vi "output.vi"(8 "error in":errorcluster, 10 "data table in":T1, 11 "UI Reference runtime in":refnum<class "io runtime.lvclass">) -> (0 "error out":errorcluster, 2 "data table out":T1, 3 "UI Reference runtime out":refnum<class "io runtime.lvclass">)   [LabVIEW 2015, in "io runtime.lvclass"]
doc: "Provides an interface for writing data to a module at runtime. While this interface performs no operations, a child should provide an override which may write to any open sessions, references, or interfaces."
uses:
  io runtime.lvclass
  <vilib>/NI/Tag Bus/table/data table.ctl
  io runtime.lvclass/io runtime.ctl
  FXP I_20_5.ctl
  FXP I_24_5.ctl
  FXP I_24_10.ctl
  <vilib>/NI/Tag Bus/table/data polymorphs/read many/read Doubles.vi
  <vilib>/NI/Tag Bus/table/data polymorphs/read many/read Singles.vi
  <vilib>/NI/Tag Bus/table/data polymorphs/read many/read I64s.vi
  <vilib>/NI/Tag Bus/table/data polymorphs/read many/read I32s.vi
  <vilib>/NI/Tag Bus/table/data polymorphs/read many/read I16s.vi
  <vilib>/NI/Tag Bus/table/data polymorphs/read many/read I8s.vi
  <vilib>/NI/Tag Bus/table/data polymorphs/read many/read U64s.vi
  <vilib>/NI/Tag Bus/table/data polymorphs/read many/read U32s.vi
  <vilib>/NI/Tag Bus/table/data polymorphs/read many/read U16s.vi
  <vilib>/NI/Tag Bus/table/data polymorphs/read many/read U8s.vi
  <vilib>/NI/Tag Bus/table/data polymorphs/read many/read Booleans.vi
  <vilib>/NI/Tag Bus/table/data polymorphs/read many/read Array of Booleans.vi
  <vilib>/NI/Tag Bus/table/data polymorphs/read one/read Array of Double.vi
  <vilib>/NI/Tag Bus/table/data polymorphs/read one/read Array of Single.vi
  <vilib>/NI/Tag Bus/table/data polymorphs/read one/read Array of I64.vi
  <vilib>/NI/Tag Bus/table/data polymorphs/read one/read Array of I32.vi
  <vilib>/NI/Tag Bus/table/data polymorphs/read one/read Array of I16.vi
  <vilib>/NI/Tag Bus/table/data polymorphs/read one/read Array of I8.vi
  <vilib>/NI/Tag Bus/table/data polymorphs/read one/read Array of U64.vi
  <vilib>/NI/Tag Bus/table/data polymorphs/read one/read Array of U32.vi
  <vilib>/NI/Tag Bus/table/data polymorphs/read one/read Array of U16.vi
  <vilib>/NI/Tag Bus/table/data polymorphs/read one/read Array of U8.vi
  <vilib>/rvi/errors/niLvFpgaAdjustHostInterfaceError.vi
  <vilib>/Utility/error.llb/Error Cluster From Error Code.vi
  <vilib>/rvi/interface/nirviReadWriteControl/nirviReadWriteControl.xnode
  <vilib>/NI/Tag Bus/table/data table.lvlib
  NiFpgaLv.dll
  <vilib>/rvi/interface/Simulation/niFpgaSimulationCallBeginRW.vi
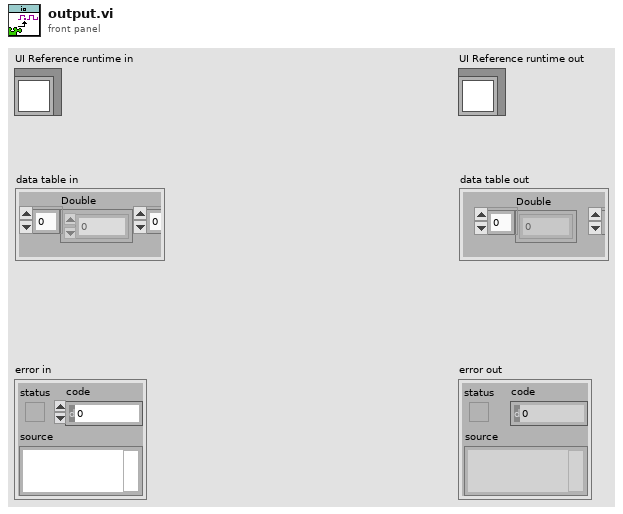
[diagram p1: front panel]
types:
  T1 = typedef "tag bus.lvlib/data table.lvlib/data table.ctl" = cluster{"Double":dbl[], "Single":sgl[], "I64":i64[], "I32":i32[], "I16":i16[], "I8":i8[], "U64":u64[], "U32":u32[], "U16":u16[], "U8":u8[], "Boolean":bool[], "String":string[], "Array of Double":cluster{"DBL Array":dbl[]}[], "Array of Single":cluster{"SGL Array":sgl[]}[], "Array of I64":cluster{"I64 Array":i64[]}[], "Array of I32":cluster{"I32 Array":i32[]}[], "Array of I16":cluster{"I16 Array":i16[]}[], "Array of I8":cluster{"I8 Array":i8[]}[], "Array of U64":cluster{"U64 Array":u64[]}[], "Array of U32":cluster{"U32 Array":u32[]}[], "Array of U16":cluster{"U16 Array":u16[]}[], "Array of U8":cluster{"U8 Array":u8[]}[], "Array of Boolean":cluster{"Boolean Array":bool[]}[], "Array of String":cluster{"String Array":string[]}[]}
  T2 = typedef "io runtime.lvclass/control index set.ctl" = cluster{"data type":T3, "fpga res type":T4[], "fpga resource":refnum<k20>[], "data indexes":i32[], "fifo timeout":refnum<k20>[], "fifo reset":refnum<k20>[], "fifo average":i32[], "fifo samples":u32[], "fifo channels":u32[]}
  T3 = typedef "tag bus.lvlib/tag descriptor.lvclass/Data Type.ctl" = enum16{"Double", "Single", "I64", "I32", "I16", "I8", "U64", "U32", "U16", "U8", "Boolean", "String", "Array of Double", "Array of Single", "Array of I64", "Array of I32", "Array of I16", "Array of I8", "Array of U64", "Array of U32", "Array of U16", "Array of U8", "Array of Boolean", "Array of String"}
  T4 = typedef "io configuration.lvclass/fpga resource supported data types.ctl" = enum16{"Invalid Type", "Single", "I64", "I32", "I16", "I8", "U64", "U32", "U16", "U8", "Boolean", "FXP I,20,5", "FXP I,24,5", "FXP I,24,10", "Fifo 1023,I16"}
  T5 = typedef "io runtime.lvclass/FXP I_20_5.ctl" = refnum<k20>
  T6 = typedef "io runtime.lvclass/FXP I_24_5.ctl" = refnum<k20>
  T7 = typedef "io runtime.lvclass/FXP I_24_10.ctl" = refnum<k20>
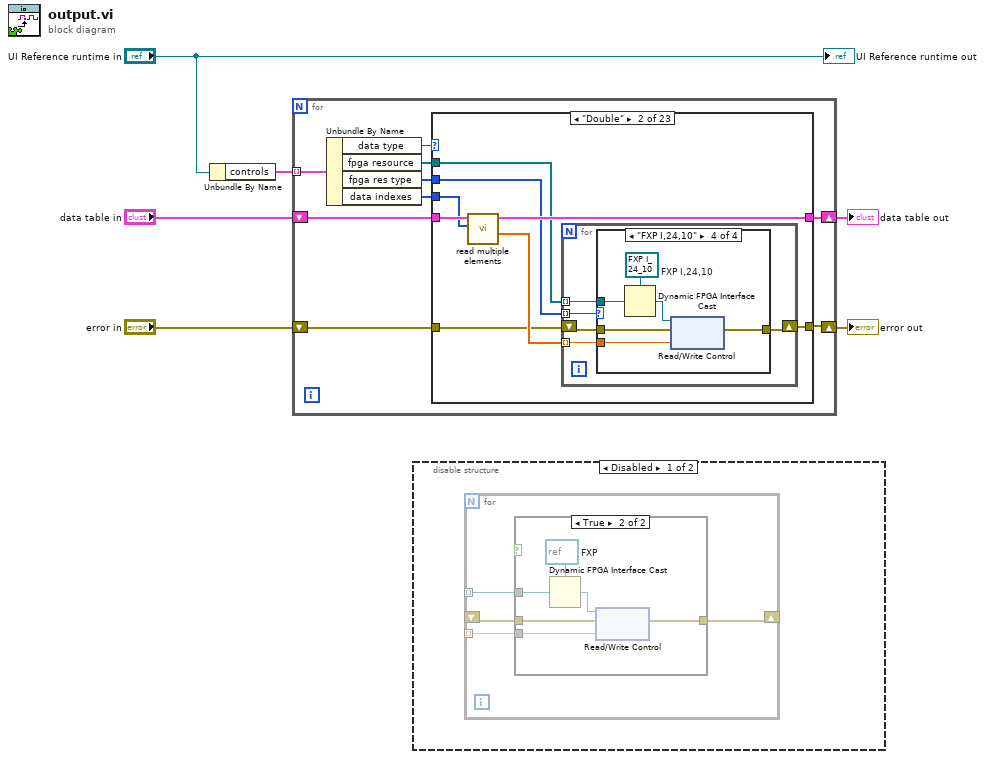
[diagram p0: block diagram]
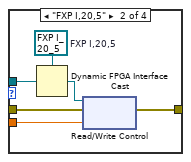
[diagram p6: hidden frame]
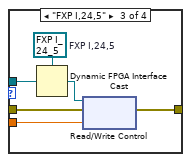
[diagram p7: hidden frame]
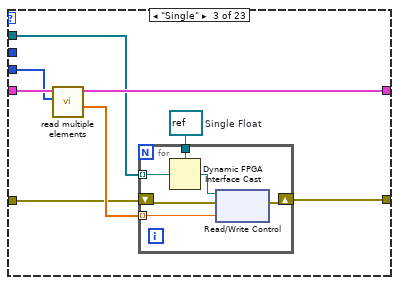
[diagram p8: hidden frame]
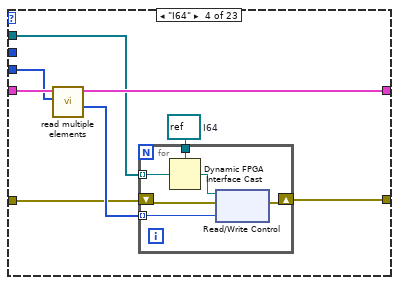
[diagram p9: hidden frame]
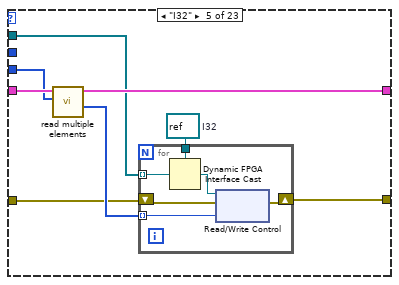
[diagram p10: hidden frame]
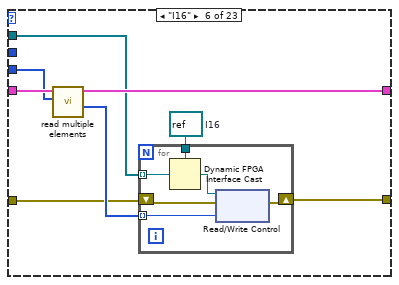
[diagram p11: hidden frame]
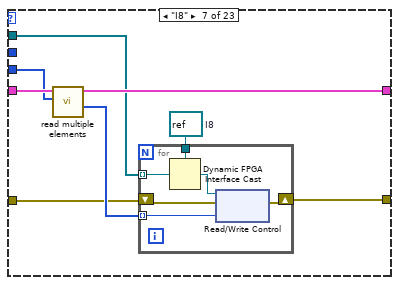
[diagram p12: hidden frame]
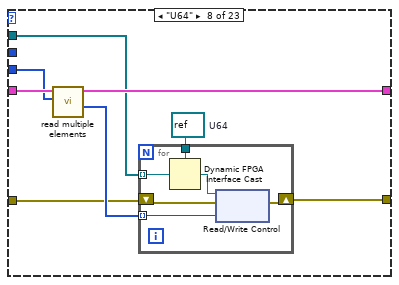
[diagram p13: hidden frame]
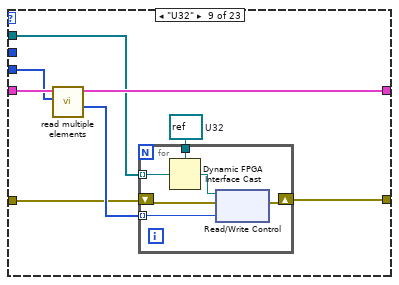
[diagram p14: hidden frame]
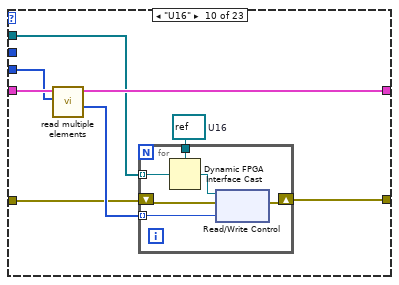
[diagram p15: hidden frame]
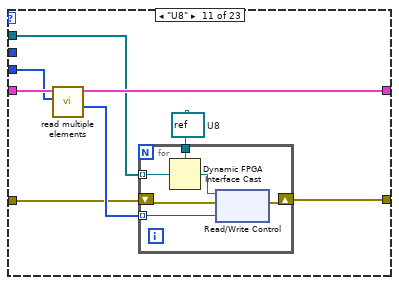
[diagram p16: hidden frame]
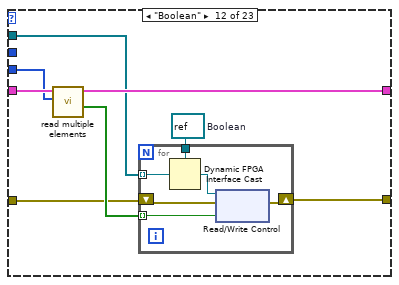
[diagram p17: hidden frame]
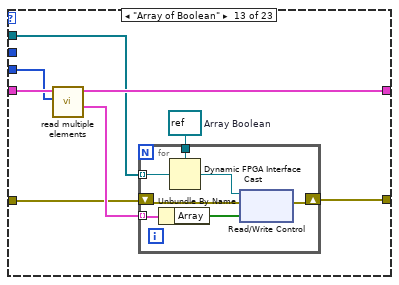
[diagram p18: hidden frame]
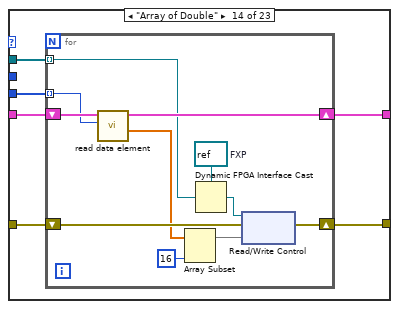
[diagram p19: hidden frame]
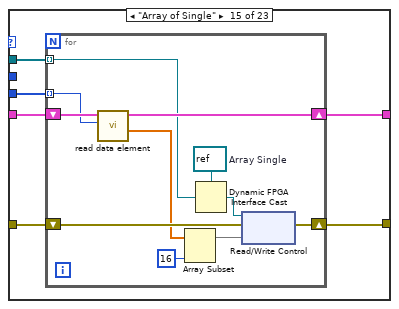
[diagram p20: hidden frame]
diagram:
  n1 = Unbundle By Name("UI Reference runtime in") -> ("controls"=w6:T2[])
  n2 = for {
    shift-right: [w14] -> w2
    shift-left: "data table in" -> [w13]
    shift-right: [w9] -> w4
    shift-left: "error in" -> [w12]
    tunnel: w6 -> [w15] mode=indexing
    n3 = Unbundle By Name(w15) -> ("data type"=w8:T3, "fpga resource"=w10:refnum<k20>[], "fpga res type"=w7:T4[], "data indexes"=w11:i32[])
    n4 = case shown="\"Double\"" w8 {
      tunnel: [w17 w24 w56 w70 w84 w98 w112 w126 w140 w154 w168 w182 w196 w209 w226 w243 w260 w276 w293 w310 w327 w344 w361] -> w14
      tunnel: w13 -> [w17 w25 w57 w71 w85 w99 w113 w127 w141 w155 w169 w183 w197 w210 w227 w244 w261 w277 w294 w311 w328 w345 w362]
      tunnel: w12 -> [w16 w21 w53 w67 w81 w95 w109 w123 w137 w151 w165 w179 w193 w207 w224 w241 w258 w274 w291 w308 w325 w342 w359]
      tunnel: w11 -> [_ w23 w55 w69 w83 w97 w111 w125 w139 w153 w167 w181 w195 w208 w225 w242 w259 w275 w292 w309 w326 w343 w360]
      tunnel: w10 -> [_ w20 w52 w66 w80 w94 w108 w122 w136 w150 w164 w178 w192 w206 w223 w240 w257 w273 w290 w307 w324 w341 w358]
      tunnel: [w16 w19 w50 w64 w78 w92 w106 w120 w134 w148 w162 w176 w191 w205 w222 w239 w256 w272 w289 w306 w323 w340 w357] -> w9
      tunnel: w7 -> [_ w18 _ _ _ _ _ _ _ _ _ _ _ _ _ _ _ _ _ _ _ _ _]
      frame Default {
      }
      frame "Double" {
        n5 = call-poly <vilib>:"read multiple elements.vi"("indices"=w23, "data table in"=w25) -> ("values"=w22:dbl[], "data table out"=w24:T1)  [unwired: 8 in]
        n6 = for {
          tunnel: w20 -> [w30] mode=indexing
          shift-right: [w28] -> w19
          shift-left: w21 -> [w29]
          tunnel: w22 -> [w27] mode=indexing
          tunnel: w18 -> [w26] mode=indexing
          n7 = case shown="\"FXP I,24,10\"" w26 {
            tunnel: w30 -> [_ w37 w43 w49]
            tunnel: w29 -> [w31 w35 w41 w47]
            tunnel: [w31 w34 w40 w46] -> w28
            tunnel: w27 -> [_ w33 w39 w45]
            frame "Invalid Type", Default {
            }
            frame "FXP I,20,5" {
              w32 = T5 refnum  # FXP I,20,5
              n8 = Dynamic FPGA Interface Cast(Session In=w32, Type=w37) -> (Session Out=w36:T5)
              n9 = xnode "Read/Write Control"("FPGA VI Reference In"=w36, "error in"=w35, "Value"=w33) -> ("error out"=w34:errorcluster)  [unwired: 1 out]
            }
            frame "FXP I,24,5" {
              w38 = T6 refnum  # FXP I,24,5
              n10 = Dynamic FPGA Interface Cast(Session In=w38, Type=w43) -> (Session Out=w42:T6)
              n11 = xnode "Read/Write Control"("FPGA VI Reference In"=w42, "error in"=w41, "Value"=w39) -> ("error out"=w40:errorcluster)  [unwired: 1 out]
            }
            frame "FXP I,24,10" {
              w44 = T7 refnum  # FXP I,24,10
              n12 = Dynamic FPGA Interface Cast(Session In=w44, Type=w49) -> (Session Out=w48:T7)
              n13 = xnode "Read/Write Control"("FPGA VI Reference In"=w48, "error in"=w47, "Value"=w45) -> ("error out"=w46:errorcluster)  [unwired: 1 out]
            }
          }
        }
      }
      frame "Single" {
        w51 = refnum<k20> refnum  # Single Float
        n14 = call-poly <vilib>:"read multiple elements.vi"("indices"=w55, "data table in"=w57) -> ("values"=w54:sgl[], "data table out"=w56:T1)  [unwired: 8 in]
        n15 = for {
          tunnel: w52 -> [w63] mode=indexing
          shift-right: [w60] -> w50
          shift-left: w53 -> [w61]
          tunnel: w51 -> [w59]
          tunnel: w54 -> [w58] mode=indexing
          n16 = Dynamic FPGA Interface Cast(Session In=w59, Type=w63) -> (Session Out=w62:refnum<k20>)
          n17 = xnode "Read/Write Control"("FPGA VI Reference In"=w62, "error in"=w61, "Value"=w58) -> ("error out"=w60:errorcluster)  [unwired: 1 out]
        }
      }
      frame "I64" {
        w65 = refnum<k20> refnum  # I64
        n18 = call-poly <vilib>:"read multiple elements.vi"("indices"=w69, "data table in"=w71) -> ("values"=w68:i64[], "data table out"=w70:T1)  [unwired: 8 in]
        n19 = for {
          tunnel: w66 -> [w77] mode=indexing
          shift-right: [w74] -> w64
          shift-left: w67 -> [w75]
          tunnel: w65 -> [w73]
          tunnel: w68 -> [w72] mode=indexing
          n20 = Dynamic FPGA Interface Cast(Session In=w73, Type=w77) -> (Session Out=w76:refnum<k20>)
          n21 = xnode "Read/Write Control"("FPGA VI Reference In"=w76, "error in"=w75, "Value"=w72) -> ("error out"=w74:errorcluster)  [unwired: 1 out]
        }
      }
      frame "I32" {
        w79 = refnum<k20> refnum  # I32
        n22 = call-poly <vilib>:"read multiple elements.vi"("indices"=w83, "data table in"=w85) -> ("values"=w82:i32[], "data table out"=w84:T1)  [unwired: 8 in]
        n23 = for {
          tunnel: w80 -> [w91] mode=indexing
          shift-right: [w88] -> w78
          shift-left: w81 -> [w89]
          tunnel: w79 -> [w87]
          tunnel: w82 -> [w86] mode=indexing
          n24 = Dynamic FPGA Interface Cast(Session In=w87, Type=w91) -> (Session Out=w90:refnum<k20>)
          n25 = xnode "Read/Write Control"("FPGA VI Reference In"=w90, "error in"=w89, "Value"=w86) -> ("error out"=w88:errorcluster)  [unwired: 1 out]
        }
      }
      frame "I16" {
        w93 = refnum<k20> refnum  # I16
        n26 = call-poly <vilib>:"read multiple elements.vi"("indices"=w97, "data table in"=w99) -> ("values"=w96:i16[], "data table out"=w98:T1)  [unwired: 8 in]
        n27 = for {
          tunnel: w94 -> [w105] mode=indexing
          shift-right: [w102] -> w92
          shift-left: w95 -> [w103]
          tunnel: w93 -> [w101]
          tunnel: w96 -> [w100] mode=indexing
          n28 = Dynamic FPGA Interface Cast(Session In=w101, Type=w105) -> (Session Out=w104:refnum<k20>)
          n29 = xnode "Read/Write Control"("FPGA VI Reference In"=w104, "error in"=w103, "Value"=w100) -> ("error out"=w102:errorcluster)  [unwired: 1 out]
        }
      }
      frame "I8" {
        w107 = refnum<k20> refnum  # I8
        n30 = call-poly <vilib>:"read multiple elements.vi"("indices"=w111, "data table in"=w113) -> ("values"=w110:i8[], "data table out"=w112:T1)  [unwired: 8 in]
        n31 = for {
          tunnel: w108 -> [w119] mode=indexing
          shift-right: [w116] -> w106
          shift-left: w109 -> [w117]
          tunnel: w107 -> [w115]
          tunnel: w110 -> [w114] mode=indexing
          n32 = Dynamic FPGA Interface Cast(Session In=w115, Type=w119) -> (Session Out=w118:refnum<k20>)
          n33 = xnode "Read/Write Control"("FPGA VI Reference In"=w118, "error in"=w117, "Value"=w114) -> ("error out"=w116:errorcluster)  [unwired: 1 out]
        }
      }
      frame "U64" {
        w121 = refnum<k20> refnum  # U64
        n34 = call-poly <vilib>:"read multiple elements.vi"("indices"=w125, "data table in"=w127) -> ("values"=w124:u64[], "data table out"=w126:T1)  [unwired: 8 in]
        n35 = for {
          tunnel: w122 -> [w133] mode=indexing
          shift-right: [w130] -> w120
          shift-left: w123 -> [w131]
          tunnel: w121 -> [w129]
          tunnel: w124 -> [w128] mode=indexing
          n36 = Dynamic FPGA Interface Cast(Session In=w129, Type=w133) -> (Session Out=w132:refnum<k20>)
          n37 = xnode "Read/Write Control"("FPGA VI Reference In"=w132, "error in"=w131, "Value"=w128) -> ("error out"=w130:errorcluster)  [unwired: 1 out]
        }
      }
      frame "U32" {
        w135 = refnum<k20> refnum  # U32
        n38 = call-poly <vilib>:"read multiple elements.vi"("indices"=w139, "data table in"=w141) -> ("values"=w138:u32[], "data table out"=w140:T1)  [unwired: 8 in]
        n39 = for {
          tunnel: w136 -> [w147] mode=indexing
          shift-right: [w144] -> w134
          shift-left: w137 -> [w145]
          tunnel: w135 -> [w143]
          tunnel: w138 -> [w142] mode=indexing
          n40 = Dynamic FPGA Interface Cast(Session In=w143, Type=w147) -> (Session Out=w146:refnum<k20>)
          n41 = xnode "Read/Write Control"("FPGA VI Reference In"=w146, "error in"=w145, "Value"=w142) -> ("error out"=w144:errorcluster)  [unwired: 1 out]
        }
      }
      frame "U16" {
        w149 = refnum<k20> refnum  # U16
        n42 = call-poly <vilib>:"read multiple elements.vi"("indices"=w153, "data table in"=w155) -> ("values"=w152:u16[], "data table out"=w154:T1)  [unwired: 8 in]
        n43 = for {
          tunnel: w150 -> [w161] mode=indexing
          shift-right: [w158] -> w148
          shift-left: w151 -> [w159]
          tunnel: w149 -> [w157]
          tunnel: w152 -> [w156] mode=indexing
          n44 = Dynamic FPGA Interface Cast(Session In=w157, Type=w161) -> (Session Out=w160:refnum<k20>)
          n45 = xnode "Read/Write Control"("FPGA VI Reference In"=w160, "error in"=w159, "Value"=w156) -> ("error out"=w158:errorcluster)  [unwired: 1 out]
        }
      }
      frame "U8" {
        w163 = refnum<k20> refnum  # U8
        n46 = call-poly <vilib>:"read multiple elements.vi"("indices"=w167, "data table in"=w169) -> ("values"=w166:u8[], "data table out"=w168:T1)  [unwired: 8 in]
        n47 = for {
          tunnel: w164 -> [w175] mode=indexing
          shift-right: [w172] -> w162
          shift-left: w165 -> [w173]
          tunnel: w163 -> [w171]
          tunnel: w166 -> [w170] mode=indexing
          n48 = Dynamic FPGA Interface Cast(Session In=w171, Type=w175) -> (Session Out=w174:refnum<k20>)
          n49 = xnode "Read/Write Control"("FPGA VI Reference In"=w174, "error in"=w173, "Value"=w170) -> ("error out"=w172:errorcluster)  [unwired: 1 out]
        }
      }
      frame "Boolean" {
        w177 = refnum<k20> refnum  # Boolean
        n50 = call-poly <vilib>:"read multiple elements.vi"("indices"=w181, "data table in"=w183) -> ("values"=w180:bool[], "data table out"=w182:T1)  [unwired: 8 in]
        n51 = for {
          tunnel: w178 -> [w189] mode=indexing
          shift-right: [w186] -> w176
          shift-left: w179 -> [w187]
          tunnel: w177 -> [w185]
          tunnel: w180 -> [w184] mode=indexing
          n52 = Dynamic FPGA Interface Cast(Session In=w185, Type=w189) -> (Session Out=w188:refnum<k20>)
          n53 = xnode "Read/Write Control"("FPGA VI Reference In"=w188, "error in"=w187, "Value"=w184) -> ("error out"=w186:errorcluster)  [unwired: 1 out]
        }
      }
      frame "Array of Boolean" {
        w190 = refnum<k20> refnum  # Array Boolean
        n54 = call-poly <vilib>:"read multiple elements.vi"("indices"=w195, "data table in"=w197) -> ("values"=w194:cluster{"Array":bool[]}[], "data table out"=w196:T1)  [unwired: 8 in]
        n55 = for {
          tunnel: w192 -> [w204] mode=indexing
          shift-right: [w201] -> w191
          shift-left: w193 -> [w202]
          tunnel: w190 -> [w200]
          tunnel: w194 -> [w199] mode=indexing
          n56 = Unbundle By Name(w199) -> ("Array"=w198:bool[])
          n57 = Dynamic FPGA Interface Cast(Session In=w200, Type=w204) -> (Session Out=w203:refnum<k20>)
          n58 = xnode "Read/Write Control"("FPGA VI Reference In"=w203, "error in"=w202, "Value"=w198) -> ("error out"=w201:errorcluster)  [unwired: 1 out]
        }
      }
      frame "Array of Double" {
        n59 = for {
          tunnel: w208 -> [w219] mode=indexing
          shift-right: [w220] -> w209
          shift-left: w210 -> [w221]
          tunnel: w206 -> [w215] mode=indexing
          shift-right: [w214] -> w205
          shift-left: w207 -> [w217]
          w216 = refnum<k20> refnum  # FXP
          n60 = call-poly <vilib>:"read data element.vi"("index"=w219, "data table in"=w221) -> ("value"=w213:dbl[], "data table out"=w220:T1)  [unwired: 8 in]
          n61 = Array Subset(array=w213, length=16) -> (w212:dbl[])  [unwired: 1 in]
          n62 = Dynamic FPGA Interface Cast(Session In=w216, Type=w215) -> (Session Out=w218:refnum<k20>)
          n63 = xnode "Read/Write Control"("FPGA VI Reference In"=w218, "error in"=w217, "Value"=w212) -> ("error out"=w214:errorcluster)  [unwired: 1 out]
        }
      }
      frame "Array of Single" {
        n64 = for {
          tunnel: w225 -> [w236] mode=indexing
          shift-right: [w237] -> w226
          shift-left: w227 -> [w238]
          tunnel: w223 -> [w233] mode=indexing
          shift-right: [w232] -> w222
          shift-left: w224 -> [w234]
          w230 = refnum<k20> refnum  # Array Single
          n65 = call-poly <vilib>:"read data element.vi"("index"=w236, "data table in"=w238) -> ("value"=w229:sgl[], "data table out"=w237:T1)  [unwired: 8 in]
          n66 = Array Subset(array=w229, length=16) -> (w228:sgl[])  [unwired: 1 in]
          n67 = Dynamic FPGA Interface Cast(Session In=w230, Type=w233) -> (Session Out=w235:refnum<k20>)
          n68 = xnode "Read/Write Control"("FPGA VI Reference In"=w235, "error in"=w234, "Value"=w228) -> ("error out"=w232:errorcluster)  [unwired: 1 out]
        }
      }
      frame "Array of I64" {
        n69 = for {
          tunnel: w242 -> [w253] mode=indexing
          shift-right: [w254] -> w243
          shift-left: w244 -> [w255]
          tunnel: w240 -> [w250] mode=indexing
          shift-right: [w249] -> w239
          shift-left: w241 -> [w251]
          w245 = refnum<k20> refnum  # Array I64
          n70 = call-poly <vilib>:"read data element.vi"("index"=w253, "data table in"=w255) -> ("value"=w248:i64[], "data table out"=w254:T1)  [unwired: 8 in]
          n71 = Array Subset(array=w248, length=16) -> (w247:i64[])  [unwired: 1 in]
          n72 = Dynamic FPGA Interface Cast(Session In=w245, Type=w250) -> (Session Out=w252:refnum<k20>)
          n73 = xnode "Read/Write Control"("FPGA VI Reference In"=w252, "error in"=w251, "Value"=w247) -> ("error out"=w249:errorcluster)  [unwired: 1 out]
        }
      }
      frame "Array of I32" {
        n74 = for {
          tunnel: w259 -> [w269] mode=indexing
          shift-right: [w270] -> w260
          shift-left: w261 -> [w271]
          tunnel: w257 -> [w266] mode=indexing
          shift-right: [w265] -> w256
          shift-left: w258 -> [w267]
          w262 = refnum<k20> refnum  # Array I32
          n75 = call-poly <vilib>:"read data element.vi"("index"=w269, "data table in"=w271) -> ("value"=w264:i32[], "data table out"=w270:T1)  [unwired: 8 in]
          n76 = Array Subset(array=w264, length=16) -> ()  [unwired: 1 in, 1 out]
          n77 = Dynamic FPGA Interface Cast(Session In=w262, Type=w266) -> (Session Out=w268:refnum<k20>)
          n78 = xnode "Read/Write Control"("FPGA VI Reference In"=w268, "error in"=w267) -> ("error out"=w265:errorcluster)  [unwired: 1 in, 1 out]
        }
      }
      frame "Array of I16" {
        n79 = for {
          tunnel: w275 -> [w286] mode=indexing
          shift-right: [w287] -> w276
          shift-left: w277 -> [w288]
          tunnel: w273 -> [w283] mode=indexing
          shift-right: [w282] -> w272
          shift-left: w274 -> [w284]
          w279 = refnum<k20> refnum  # Array I16
          n80 = call-poly <vilib>:"read data element.vi"("index"=w286, "data table in"=w288) -> ("value"=w281:i16[], "data table out"=w287:T1)  [unwired: 8 in]
          n81 = Array Subset(array=w281, length=16) -> (w278:i16[])  [unwired: 1 in]
          n82 = Dynamic FPGA Interface Cast(Session In=w279, Type=w283) -> (Session Out=w285:refnum<k20>)
          n83 = xnode "Read/Write Control"("FPGA VI Reference In"=w285, "error in"=w284, "Value"=w278) -> ("error out"=w282:errorcluster)  [unwired: 1 out]
        }
      }
      frame "Array of I8" {
        n84 = for {
          tunnel: w292 -> [w303] mode=indexing
          shift-right: [w304] -> w293
          shift-left: w294 -> [w305]
          tunnel: w290 -> [w300] mode=indexing
          shift-right: [w299] -> w289
          shift-left: w291 -> [w301]
          w295 = refnum<k20> refnum  # Array I8
          n85 = call-poly <vilib>:"read data element.vi"("index"=w303, "data table in"=w305) -> ("value"=w298:i8[], "data table out"=w304:T1)  [unwired: 8 in]
          n86 = Array Subset(array=w298, length=16) -> (w296:i8[])  [unwired: 1 in]
          n87 = Dynamic FPGA Interface Cast(Session In=w295, Type=w300) -> (Session Out=w302:refnum<k20>)
          n88 = xnode "Read/Write Control"("FPGA VI Reference In"=w302, "error in"=w301, "Value"=w296) -> ("error out"=w299:errorcluster)  [unwired: 1 out]
        }
      }
      frame "Array of U64" {
        n89 = for {
          tunnel: w309 -> [w320] mode=indexing
          shift-right: [w321] -> w310
          shift-left: w311 -> [w322]
          tunnel: w307 -> [w317] mode=indexing
          shift-right: [w316] -> w306
          shift-left: w308 -> [w318]
          w312 = refnum<k20> refnum  # Array U64
          n90 = call-poly <vilib>:"read data element.vi"("index"=w320, "data table in"=w322) -> ("value"=w315:u64[], "data table out"=w321:T1)  [unwired: 8 in]
          n91 = Array Subset(array=w315, length=16) -> (w313:u64[])  [unwired: 1 in]
          n92 = Dynamic FPGA Interface Cast(Session In=w312, Type=w317) -> (Session Out=w319:refnum<k20>)
          n93 = xnode "Read/Write Control"("FPGA VI Reference In"=w319, "error in"=w318, "Value"=w313) -> ("error out"=w316:errorcluster)  [unwired: 1 out]
        }
      }
      frame "Array of U32" {
        n94 = for {
          tunnel: w326 -> [w337] mode=indexing
          shift-right: [w338] -> w327
          shift-left: w328 -> [w339]
          tunnel: w324 -> [w334] mode=indexing
          shift-right: [w333] -> w323
          shift-left: w325 -> [w335]
          w329 = refnum<k20> refnum  # Array U32
          n95 = call-poly <vilib>:"read data element.vi"("index"=w337, "data table in"=w339) -> ("value"=w332:u32[], "data table out"=w338:T1)  [unwired: 8 in]
          n96 = Array Subset(array=w332, length=16) -> (w330:u32[])  [unwired: 1 in]
          n97 = Dynamic FPGA Interface Cast(Session In=w329, Type=w334) -> (Session Out=w336:refnum<k20>)
          n98 = xnode "Read/Write Control"("FPGA VI Reference In"=w336, "error in"=w335, "Value"=w330) -> ("error out"=w333:errorcluster)  [unwired: 1 out]
        }
      }
      frame "Array of U16" {
        n99 = for {
          tunnel: w343 -> [w354] mode=indexing
          shift-right: [w355] -> w344
          shift-left: w345 -> [w356]
          tunnel: w341 -> [w351] mode=indexing
          shift-right: [w350] -> w340
          shift-left: w342 -> [w352]
          w346 = refnum<k20> refnum  # Array U16
          n100 = call-poly <vilib>:"read data element.vi"("index"=w354, "data table in"=w356) -> ("value"=w349:u16[], "data table out"=w355:T1)  [unwired: 8 in]
          n101 = Array Subset(array=w349, length=16) -> (w347:u16[])  [unwired: 1 in]
          n102 = Dynamic FPGA Interface Cast(Session In=w346, Type=w351) -> (Session Out=w353:refnum<k20>)
          n103 = xnode "Read/Write Control"("FPGA VI Reference In"=w353, "error in"=w352, "Value"=w347) -> ("error out"=w350:errorcluster)  [unwired: 1 out]
        }
      }
      frame "Array of U8" {
        n104 = for {
          tunnel: w360 -> [w371] mode=indexing
          shift-right: [w372] -> w361
          shift-left: w362 -> [w373]
          tunnel: w358 -> [w368] mode=indexing
          shift-right: [w367] -> w357
          shift-left: w359 -> [w369]
          w363 = refnum<k20> refnum  # Array U8
          n105 = call-poly <vilib>:"read data element.vi"("index"=w371, "data table in"=w373) -> ("value"=w366:u8[], "data table out"=w372:T1)  [unwired: 8 in]
          n106 = Array Subset(array=w366, length=16) -> (w364:u8[])  [unwired: 1 in]
          n107 = Dynamic FPGA Interface Cast(Session In=w363, Type=w368) -> (Session Out=w370:refnum<k20>)
          n108 = xnode "Read/Write Control"("FPGA VI Reference In"=w370, "error in"=w369, "Value"=w364) -> ("error out"=w367:errorcluster)  [unwired: 1 out]
        }
      }
    }
  }
  "error out" <- w4
  "data table out" <- w2
  n109 = disable-structure shown="Disabled" {
    frame Disabled {
      n110 = for {
        tunnel: _ -> [w378] mode=indexing
        shift-right: [w376] -> w374
        shift-left: _ -> [w377]
        tunnel: _ -> [w375] mode=indexing
        n111 = case shown="True" {
          selector: _ -> [_ _]
          tunnel: w378 -> [_ w384]
          tunnel: w377 -> [_ w382]
          tunnel: [_ w381] -> w376
          tunnel: w375 -> [_ w380]
          frame False {
          }
          frame True {
            w379 = refnum<k20> refnum  # FXP
            n112 = Dynamic FPGA Interface Cast(Session In=w379) -> (Type=w384:refnum<k20>, Session Out=w383:refnum<k20>)
            n113 = xnode "Read/Write Control"("FPGA VI Reference In"=w383, "error in"=w382) -> ("error out"=w381:errorcluster, "Value"=w380:fxp<+,32,17>)  [unwired: 1 out]
          }
        }
      }
    }
    frame Enabled {
    }
  }
  "UI Reference runtime out" <- "UI Reference runtime in"
